vi "ResolveError.vi"(3 "error in":errorcluster) -> (0 "error out":errorcluster)   [LabVIEW 2015, in "MiscHelperVIs.lvlib"]
uses:
  MiscHelperVIs.lvlib
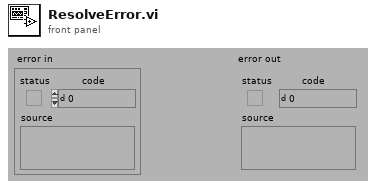
[diagram p1: front panel]
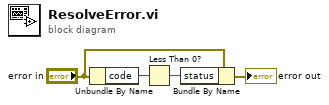
[diagram p0: block diagram]
diagram:
  n1 = Unbundle By Name("error in") -> ("code"=w2:i32)
  n2 = Less Than 0?(x=w2) -> (x < 0?=w3:bool)
  n3 = Bundle By Name(cluster="error in", "status"=w3) -> (→"error out":errorcluster)
